vi "queue sm 2.vi"() -> ()   [LabVIEW 2020]
uses:
  file I O/ASSIGN 8/que sm states.ctl
panel:
  out "State output":string
  out "state":T1
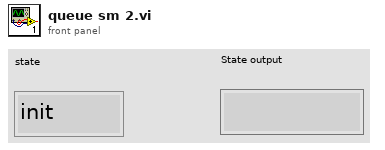
[diagram p1: front panel]
types:
  T1 = typedef "que sm states.ctl" = enum16{"init", "events", "state 1", "state 2", "stop"}
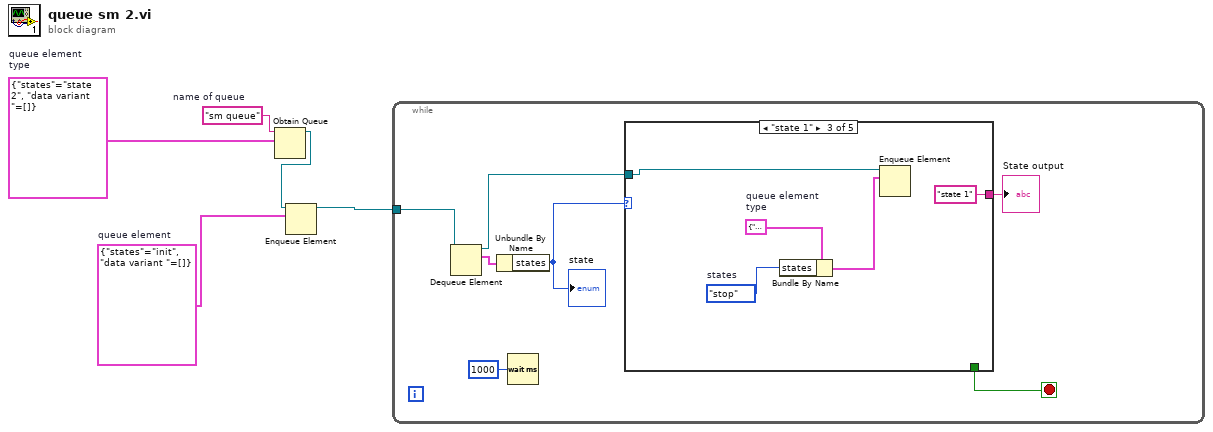
[diagram p0: block diagram]
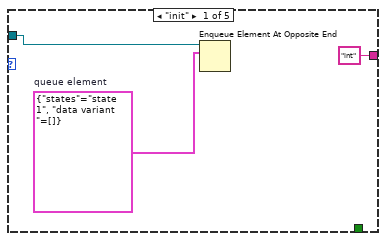
[diagram p2: hidden frame]
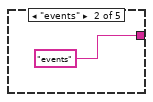
[diagram p3: hidden frame]
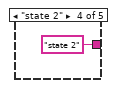
[diagram p4: hidden frame]
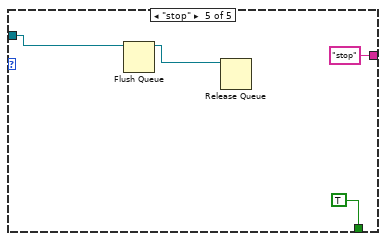
[diagram p5: hidden frame]
diagram:
  w1 = cluster{"states":T1, "data variant ":variant[]} {"states"=enum."init", "data variant "=[]}  # queue element
  w2 = cluster{"states":T1, "data variant ":variant[]} {"states"=enum."state 2", "data variant "=[]}  # queue element type
  w5 = "sm queue"  # name of queue
  n1 = Obtain Queue(name (unnamed)=w5, element data type=w2) -> (queue out=w4:refnum<queue>)  [unwired: 3 in, 2 out]
  n2 = Enqueue Element(queue=w4, element=w1) -> (queue out=w3:refnum<queue>)  [unwired: 2 in, 2 out]
  n3 = while {
    tunnel: w3 -> [w9]
    stop <- w6 stop-if-true
    n4 = Dequeue Element(queue=w9) -> (queue out=w8:refnum<queue>, element=w12:cluster{"states":T1, "data variant ":variant[]})  [unwired: 2 in, 2 out]
    n5 = Unbundle By Name(w12) -> ("states"=w7:T1)
    "state" <- w7
    n6 = Wait (ms)(milliseconds to wait=u32 1000) -> ()  [unwired: 1 out]
    n7 = case shown="\"state 1\"" w7 {
      tunnel: w8 -> [w15 _ w20 _ w24]
      tunnel: ["int" "events" "state 1" "state 2" "stop"] -> w10
      tunnel: [_ _ _ _ TRUE] -> w6
      frame "init" {
        w13 = cluster{"states":T1, "data variant ":variant[]} {"states"=enum."state 1", "data variant "=[]}  # queue element
        n8 = Enqueue Element At Opposite End(queue=w15, element=w13) -> ()  [unwired: 2 in, 3 out]
      }
      frame "events" {
      }
      frame "state 1" {
        w17 = cluster{"states":T1, "data variant ":variant[]} {"states"=enum."state 2", "data variant "=[]}  # queue element type
        w19 = que_sm_states."stop"  # states
        n9 = Bundle By Name(cluster=w17, "states"=w19) -> (w18:cluster{"states":T1, "data variant ":variant[]})
        n10 = Enqueue Element(queue=w20, element=w18) -> ()  [unwired: 2 in, 3 out]
      }
      frame "state 2" {
      }
      frame "stop" {
        n11 = Flush Queue(queue=w24) -> (queue out=w23:refnum<queue>)  [unwired: 1 in, 2 out]
        n12 = Release Queue(queue=w23) -> ()  [unwired: 2 in, 3 out]
      }
    }
    "State output" <- w10
  }
